vi "Get Name.vi"(8 "error in (no error)":errorcluster, 11 "Grab in":refnum<class "Grab.lvclass">) -> (0 "error out":errorcluster, 2 "Command Name":string, 3 "Grab out":refnum<class "Grab.lvclass">)   [LabVIEW 2014, in "Grabber.lvlib" / "Grab.lvlib" / "Grab.lvclass"]
uses:
  Grab.lvclass
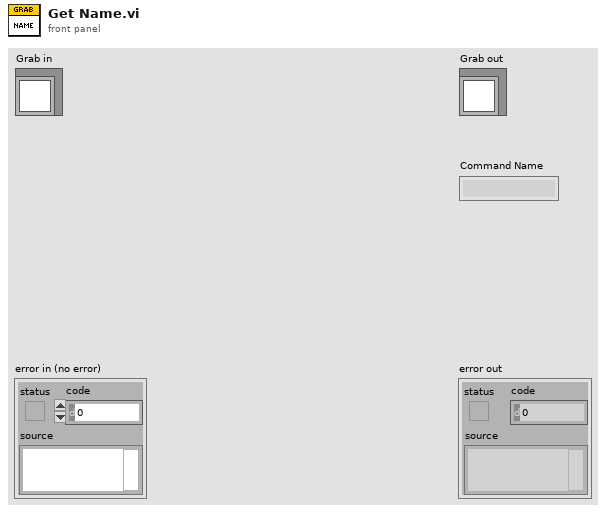
[diagram p1: front panel]
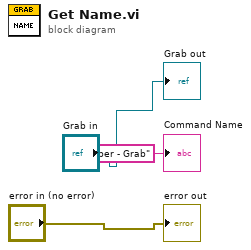
[diagram p0: block diagram]
diagram:
  "error out" <- "error in (no error)"
  "Grab out" <- "Grab in"
  "Command Name" <- "Grabber - Grab" ("Command Name")
